vi "logLowerMirrorComplete.vi"(8 "error in (no error)":errorcluster, 10 "EventLowerMirrorComplete":T1, 11 "M1M3SAL in":refnum<class "M1M3SAL.lvclass">) -> (0 "error out":errorcluster, 3 "M1M3SAL out":refnum<class "M1M3SAL.lvclass">)   [LabVIEW 2016, in "M1M3SupportCommunicator.lvlib" / "M1M3SAL.lvclass"]
uses:
  M1M3SAL.lvclass
  DataTypes/Topics/EventLowerMirrorComplete.ctl
  DataTypes/Topics/Parts/Timestamp.ctl
  DataTypes/MessageHeader.ctl
  DataTypes/MessageTypes.ctl
  DataTypes/MessageTopics.ctl
  Common_RT_Utilities/U8ArrayBuilderAutoIndexing/U8ArrayBuilderAutoIndexing.lvclass
  M1M3SupportCommunicator.lvlib
  DataTypes/Topics/M1M3SupportTopics.lvlib
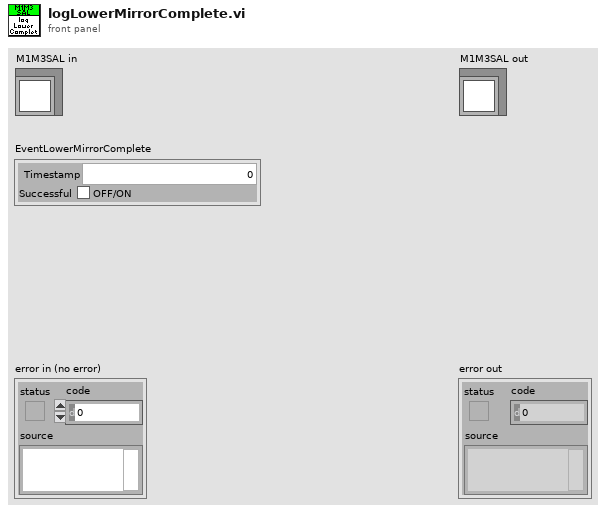
[diagram p1: front panel]
types:
  T1 = typedef "M1M3SupportTopics.lvlib/EventLowerMirrorComplete.ctl" = cluster{"Timestamp":T2, "Successful":bool}
  T2 = typedef "M1M3SupportTopics.lvlib/Timestamp.ctl" = dbl
  T3 = typedef "M1M3SupportCommunicator.lvlib/MessageHeader.ctl" = cluster{"Type":T4, "Topic":T5, "Size":i32}
  T4 = typedef "M1M3SupportCommunicator.lvlib/MessageTypes.ctl" = enum8{"None", "PutSample", "GetNextSample", "LogEvent", "GetEvent", "IssueCommand", "CommandId", "WaitForCompletion", "AcceptCommand", "AckCommand"}
  T5 = typedef "M1M3SupportCommunicator.lvlib/MessageTopics.ctl" = enum8{"None", "ForceActuatorData", "MirrorForceData", "HardpointData", "AirData", "DynamicData", "FPGAData", "IMSData", "ForceActuatorStatus", "ElevationData", "HardpointStatus", "HardpointActuatorChase", "AirStatus", "ForceActuatorSafetyChecks", "ForceActuatorTest", "ActuatorBroadcastCounter", "StatusChecks", "CellChecks", "HardpointActuatorBreakaway", "RaiseMirrorComplete", "ILCCommunication", "ElevationAngleChecks", "DetailedState", "ServoLoops", "ForceActuatorInfo", "LowerMirrorComplete", "HardpointActuatorInfo", "SettingsApplied", "ErrorCode", "StartupChecks", "SummaryState", "SettingVersions", "ActuatorTestStatus", "AppliedSettingsMatchStart", "Enable", "EnterMaintenance", "Standby", "AbortLowerM1M3", "ApplyAberrationByForces", "ApplyAOSCorrectionByBendingModes", "ClearAOSCorrection", "Start", "RaiseM1M3", "TestForceActuator", "LowerM1M3", "ApplyAOSCorrectionByForces", "Disable", "ApplyAberationByBendingMode", "TestHardpoint", "ManipulateM1M3", "ClearAberration", "Exit", "TestAir", "AbortRaiseM1M3", "MoveHardpointActuators", "ExitMaintenance", "Shutdown"}
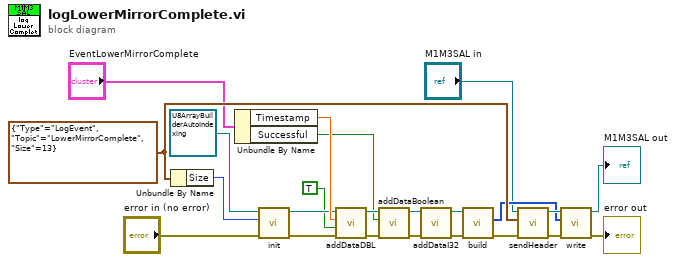
[diagram p0: block diagram]
diagram:
  w22 = T3 {"Type"=enum."LogEvent", "Topic"=enum."LowerMirrorComplete", "Size"=13} ("MessageHeader")
  n1 = Unbundle By Name(w22) -> ("Size"=w21:i32)
  n2 = Unbundle By Name("EventLowerMirrorComplete") -> ("Timestamp"=w12:T2, "Successful"=w5:bool)
  n3 = call "init.vi"("error in (no error)"="error in (no error)", "Size"=w21, "U8ArrayBuilderAutoIndexing in"=refnum<class "U8ArrayBuilderAutoIndexing.lvclass"> refnum ("RTUtilities.lvlib:U8ArrayBuilderAutoIndexing.lvclass")) -> ("error out"=w9:errorcluster, "U8ArrayBuilderAutoIndexing out"=w11:refnum<class "U8ArrayBuilderAutoIndexing.lvclass">)  [unwired: 7 in]
  n4 = call "addDataDBL.vi"("error in (no error)"=w9, "OverrideSwapBytes"=TRUE, "Data"=w12, "U8ArrayBuilderAutoIndexing in"=w11) -> ("error out"=w6:errorcluster, "U8ArrayBuilderAutoIndexing out"=w7:refnum<class "U8ArrayBuilderAutoIndexing.lvclass">)  [unwired: 6 in]
  n5 = call "addDataBoolean.vi"("error in (no error)"=w6, "Data"=w5, "U8ArrayBuilderAutoIndexing in"=w7) -> ("error out"=w3:errorcluster, "U8ArrayBuilderAutoIndexing out"=w4:refnum<class "U8ArrayBuilderAutoIndexing.lvclass">)  [unwired: 7 in]
  n6 = call "addDataI32.vi"("error in (no error)"=w3, "U8ArrayBuilderAutoIndexing in"=w4) -> ("error out"=w1:errorcluster, "U8ArrayBuilderAutoIndexing out"=w2:refnum<class "U8ArrayBuilderAutoIndexing.lvclass">)  [unwired: 8 in]
  n7 = call "build.vi"("error in (no error)"=w1, "U8ArrayBuilderAutoIndexing in"=w2) -> ("error out"=w18:errorcluster, "Array"=w19:u8[])  [unwired: 7 in, 1 out]
  n8 = call "sendHeader.vi"("error in (no error)"=w18, "MessageHeader"=w22, "M1M3SAL in"="M1M3SAL in") -> ("error out"=w17:errorcluster, "M1M3SAL out"=w20:refnum<class "M1M3SAL.lvclass">)  [unwired: 7 in]
  n9 = call "write.vi"("error in (no error)"=w17, "Data"=w19, "M1M3SAL in"=w20) -> ("error out"=→"error out":errorcluster, "M1M3SAL out"=→"M1M3SAL out":refnum<class "M1M3SAL.lvclass">)  [unwired: 7 in]
